vi "ConvertPrimitivesToIcons.vi"() -> ()   [LabVIEW 2014]
panel:
  in  "TDMS Path":path
  out "Progress":dbl(slide) scale=0.0..1.0
  out "Array":string[](array[string])
  in  "Folder Path":path=path "J:/SAPHIR/LUGE_IhmTactile/Pipboy/LabVIEW/PipBoy/needed/primitives"
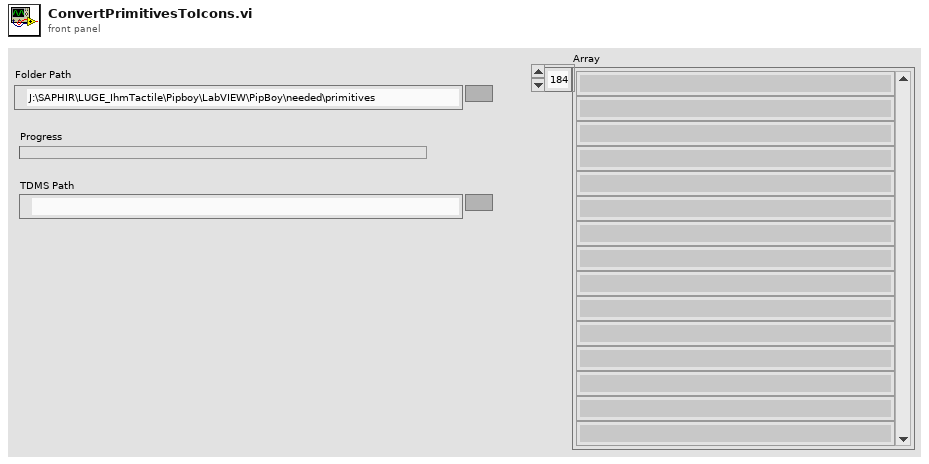
[diagram p1: front panel]
types:
  T1 = enum16{"open", "open or create", "create or replace", "create", "open (read-only)"}
  T2 = typedef "imagedata.ctl" = cluster{"image type":i32, "image depth":i32, "image":u8[], "mask":u8[], "colors":u32[], "Rectangle":cluster{"left":i16, "top":i16, "right":i16, "bottom":i16}}
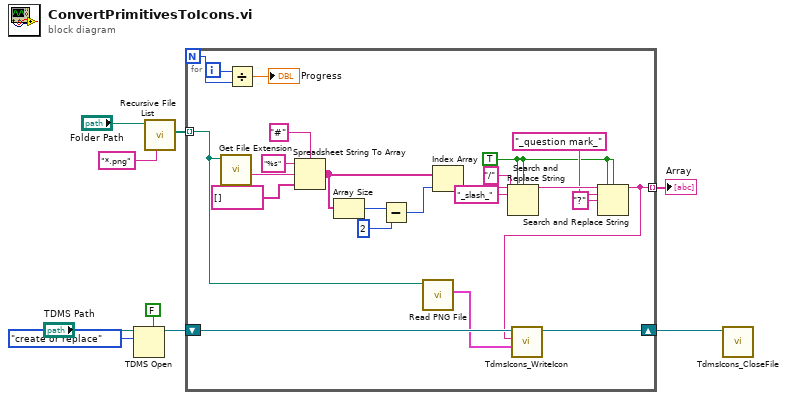
[diagram p0: block diagram]
diagram:
  n1 = TDMS Open(5:FALSE ("create index file? (T)"), 10:T1."create or replace" ("operation (0:open)"), 11:"TDMS Path") -> (3:w2:refnum<k34>)  [unwired: 4 in, 1 out]
  n2 = call <vilib>:"Recursive File List.vi"("pattern"="*.png", "Folder Path"="Folder Path") -> ("All Files in Dir"=w7:path[])  [unwired: 5 in, 4 out]
  n3 = for {
    N -> [w15]
    tunnel: w7 -> [w17] mode=indexing
    tunnel: [w11] -> w6 mode=indexing
    shift-right: [w12] -> w1
    shift-left: w2 -> [w13]
    i -> [w14]
    w18 = TRUE ("replace all? (F)")
    n4 = call <vilib>:"Get File Extension.vi"("file"=w17) -> ("filename without extension"=w32:string)  [unwired: 7 in, 3 out]
    n5 = Divide(x=w14, y=w15) -> (x/y=→"Progress":dbl)
    n6 = Spreadsheet String To Array(delimiter (Tab)="#", format string="%s", spreadsheet string=w32, array type (2D Dbl)=string[] []) -> (array=w28:string[])
    n7 = Array Size(array=w28) -> (size(s)=w27:i32)
    n8 = Subtract(x=w27, y=2) -> (x-y=w25:i32)
    n9 = call <vilib>:"Read PNG File.vi"("path to PNG file"=w17) -> ("image data"=w10:T2)  [unwired: 8 in, 2 out]
    n10 = Index Array(array=w28, index=w25) -> (element=w24:string)
    n11 = Search and Replace String(replace all?=w18, case sensitive?=w18, input string=w24, search string="_slash_", replace string="/" ("replace string (\"\")")) -> (result string=w21:string)  [unwired: 3 in, 3 out]
    n12 = Search and Replace String(replace all?=w18, case sensitive?=w18, input string=w21, search string="_question mark_", replace string="?" ("replace string (\"\")")) -> (result string=w11:string)  [unwired: 3 in, 3 out]
    n13 = call "TdmsIcons_WriteIcon.vi"("Icon"=w10, "Function"=w11, "TdmsIn"=w13) -> ("TdmsOut"=w12:refnum<k34>)  [unwired: 7 in, 1 out]
  }
  "Array" <- w6
  n14 = call "TdmsIcons_CloseFile.vi"("TdmsIn"=w1) -> ()  [unwired: 9 in, 2 out]
